vi "AI Timestamp Basics.vi"() -> ()   [LabVIEW 2020]
uses:
  <vilib>/DAQmx/write.llb/DAQmx Write (Digital Bool 1Line 1Point).vi
  <vilib>/DAQmx/read.llb/DAQmx Read (Analog Wfm 1Chan NSamp).vi
  Utility VIs/Controls/Utilities-Wait.vi/89bc9713-8f2c-40bd-a11f-1c800a437687.vi
  <vilib>/Utility/High Resolution Relative Seconds.vi
  <vilib>/DAQmx/create/channels.llb/DAQmx Create Channel (AI-Voltage-Basic).vi
  <vilib>/DAQmx/configure/timing.llb/DAQmx Timing (Sample Clock).vi
  <vilib>/DAQmx/create/channels.llb/DAQmx Create Channel (DO-Digital Output).vi
  <vilib>/Utility/High Resolution Polling Wait.vi
  <vilib>/DAQmx/miscellaneous.llb/DAQmx Fill In Error Info.vi
panel:
  out "Iteration":i32
  out "finished":bool
  out "Graph":waveform(dbl)(graph)
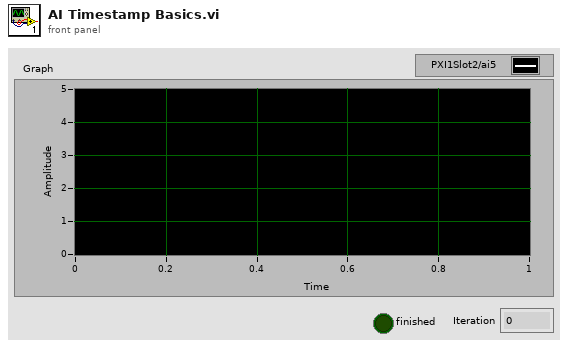
[diagram p1: front panel]
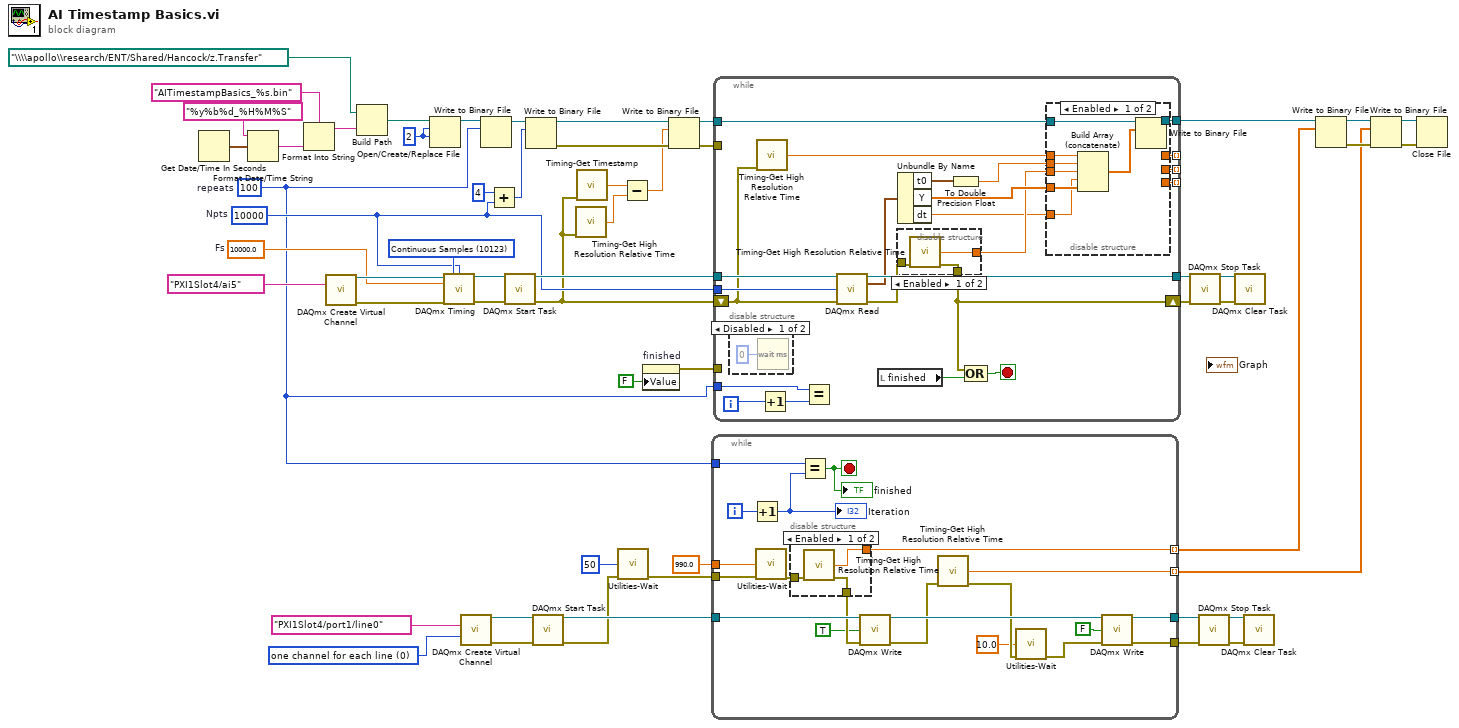
[diagram p0: block diagram]
diagram:
  w19 = 0 items=["one channel for each line", "one channel for all lines"] ("line grouping")
  w34 = u16 2
  w45 = 10000.0  # Fs
  w31 = 10000  # Npts
  w54 = 10123 items=["Finite Samples"=10178, "Continuous Samples"=10123, "Hardware Timed Single Point"=12522] ("sample mode")
  w21 = 100  # repeats
  n1 = Get Date/Time In Seconds() -> (seconds since 1Jan1904=w42:timestamp)
  n2 = Format Date/Time String(time format string (%c)="%y%b%d_%H%M%S", seconds (now)=w42) -> (date/time string=w40:string)  [unwired: 1 in]
  n3 = Format Into String(format string="AITimestampBasics_%s.bin", w40) -> (resulting string=w37:string)  [unwired: 2 in, 1 out]
  n4 = call-poly <vilib>:"DAQmx Create Virtual Channel.vi"("physical channels"=tag "PXI1Slot4/ai5") -> ("task out"=w56:refnum<k21>, "error out"=w55:errorcluster)  [unwired: 13 in]
  n5 = Build Path(base path=path "\\\\apollo\\research/ENT/Shared/Hancock/z.Transfer" ("file path (use dialog)"), name or relative path=w37) -> (appended path=w36:path)
  n6 = Open/Create/Replace File(file path (use dialog)=w36, operation (0:open)=w34, access (0:read/write)=w34) -> (refnum out=w33:refnum<file>)  [unwired: 3 in, 2 out]
  n7 = call-poly <vilib>:"DAQmx Timing.vi"("task/channels in"=w56, "sample mode"=w54, "samples per channel"=w31, "rate"=w45, "error in"=w55) -> ("task out"=w47:refnum<k21>, "error out"=w46:errorcluster)  [unwired: 9 in]
  n8 = call-poly <vilib>:"DAQmx Create Virtual Channel.vi"("lines"=tag "PXI1Slot4/port1/line0", "line grouping"=w19) -> ("task out"=w13:refnum<k21>, "error out"=w12:errorcluster)  [unwired: 12 in]
  n9 = Write to Binary File(file (use dialog)=w33, data=w21) -> (refnum out=w32:refnum<file>)  [unwired: 4 in, 2 out]
  n10 = Add(x=4, y=w31) -> (x+y=w30:i32)
  n11 = call <vilib>:"DAQmx Start Task.vi"("task/channels in"=w47, "error in"=w46) -> ("task out"=w53:refnum<k21>, "error out"=w3:errorcluster)  [unwired: 12 in]
  n12 = Write to Binary File(file (use dialog)=w32, data=w30) -> (refnum out=w27:refnum<file>, error out=w26:errorcluster)  [unwired: 4 in, 1 out]
  n13 = call <vilib>:"DAQmx Start Task.vi"("task/channels in"=w13, "error in"=w12) -> ("task out"=w14:refnum<k21>, "error out"=w10:errorcluster)  [unwired: 12 in]
  n14 = call "Timing-Get High Resolution Relative Time.vi"("error in (no error)"=w3) -> ("double precision float"=w23:dbl)  [unwired: 13 in, 1 out]
  n15 = call "Timing-Get Timestamp.vi"("error in (no error)"=w3) -> ("double precision float"=w24:dbl)  [unwired: 13 in, 1 out]
  n16 = call "Utilities-Wait.vi"("milliseconds to wait"=u32 50, "error in (no error)"=w10) -> ("error out"=w11:errorcluster)  [unwired: 13 in]
  n17 = Subtract(x=w24, y=w23) -> (x-y=w22:dbl)
  n18 = property on="finished" class="Bool (strict)"("Value"=FALSE ("finished")) -> (error out=w44:errorcluster)  [unwired: 2 in, 1 out]
  n19 = Write to Binary File(file (use dialog)=w27, data=w22, error in=w26) -> (refnum out=w28:refnum<file>, error out=w25:errorcluster)  [unwired: 3 in, 1 out]
  n20 = while {
    tunnel: w14 -> [w76]
    tunnel: [w73] -> w16
    tunnel: [w72] -> w15
    tunnel: [w70] -> w1 mode=indexing
    tunnel: w21 -> [w71]
    tunnel: [w62] -> w2 mode=indexing
    tunnel: w11 -> [w59]
    tunnel: 990.0 ("milliseconds to wait") -> [w57]
    i -> [w66]
    stop <- w67 stop-if-true
    n21 = Increment(x=w66) -> (x+1=w65:i32)
    "Iteration" <- w65
    n22 = call "Utilities-Wait.vi"("milliseconds to wait"=w57, "error in (no error)"=w59) -> ("error out"=w64:errorcluster)  [unwired: 13 in]
    n23 = disable-structure shown="Enabled" {
      disable-tunnel: w64 -> [w79 w80]
      disable-tunnel: [w78 w80] -> w63
      disable-tunnel: [w77 _] -> w62
      frame Enabled {
        n24 = call "Timing-Get High Resolution Relative Time.vi"("error in (no error)"=w79) -> ("double precision float"=w77:dbl, "error out"=w78:errorcluster)  [unwired: 13 in]
      }
      frame Disabled {
      }
    }
    n25 = Equal?(x=w71, y=w65) -> (x = y?=w67:bool)
    "finished" <- w67
    n26 = call-poly <vilib>:"DAQmx Write.vi"("task/channels in"=w76, "data"=TRUE, "error in"=w63) -> ("task out"=w75:refnum<k21>, "error out"=w69:errorcluster)  [unwired: 10 in, 1 out]
    n27 = call "Timing-Get High Resolution Relative Time.vi"("error in (no error)"=w69) -> ("double precision float"=w70:dbl, "error out"=w68:errorcluster)  [unwired: 13 in]
    n28 = call "Utilities-Wait.vi"("milliseconds to wait"=10.0, "error in (no error)"=w68) -> ("error out"=w74:errorcluster)  [unwired: 13 in]
    n29 = call-poly <vilib>:"DAQmx Write.vi"("task/channels in"=w75, "data"=FALSE, "error in"=w74) -> ("task out"=w73:refnum<k21>, "error out"=w72:errorcluster)  [unwired: 10 in, 1 out]
  }
  n30 = while {
    tunnel: w53 -> [w103]
    tunnel: [w102] -> w52
    tunnel: w31 -> [w101]
    tunnel: w44 -> [_]
    tunnel: w28 -> [w95]
    tunnel: [w94] -> w35
    tunnel: w25 -> [_]
    shift-right: [w96] -> w51
    shift-left: w3 -> [w82]
    tunnel: w21 -> [w89]
    tunnel: [w87] -> _ mode=indexing
    tunnel: [w86] -> _ mode=indexing
    tunnel: [w85] -> _ mode=indexing
    i -> [w90]
    stop <- w100 stop-if-true
    n31 = disable-structure shown="Disabled" {
      frame Disabled {
        n32 = Wait (ms)(milliseconds to wait=u32 0) -> ()  [unwired: 1 out]
      }
      frame Enabled {
      }
    }
    n33 = call "Timing-Get High Resolution Relative Time.vi"("error in (no error)"=w82) -> ("double precision float"=w81:dbl)  [unwired: 13 in, 1 out]
    n34 = Increment(x=w90) -> (x+1=w88:i32)
    n35 = Equal?(x=w89, y=w88) -> ()  [unwired: 1 out]
    n36 = call-poly <vilib>:"DAQmx Read.vi"("task/channels in"=w103, "number of samples per channel"=w101, "error in"=w82) -> ("task out"=w102:refnum<k21>, "data"=w83:waveform(dbl), "error out"=w99:errorcluster)  [unwired: 10 in]
    n37 = local read "finished"() -> (w84:bool)
    n38 = Unbundle By Name(w83) -> ("t0"=w98:timestamp, "Y"=w93:dbl[], "dt"=w91:dbl)
    n39 = disable-structure shown="Enabled" {
      disable-tunnel: w99 -> [w119 w120]
      disable-tunnel: [w118 w120] -> w96
      disable-tunnel: [w117 _] -> w92
      frame Enabled {
        n40 = call "Timing-Get High Resolution Relative Time.vi"("error in (no error)"=w119) -> ("double precision float"=w117:dbl, "error out"=w118:errorcluster)  [unwired: 13 in]
      }
      frame Disabled {
      }
    }
    n41 = To Double Precision Float(number=w98) -> (double precision float=w97:dbl)
    n42 = Compound Arithmetic op=OR(w96, w84) -> (w100:bool)
    n43 = disable-structure shown="Enabled" {
      disable-tunnel: w81 -> [w112 w115]
      disable-tunnel: w97 -> [w111 w114]
      disable-tunnel: w95 -> [w110 w116]
      disable-tunnel: [w108 w116] -> w94
      disable-tunnel: w93 -> [w107 _]
      disable-tunnel: w92 -> [w106 w113]
      disable-tunnel: w91 -> [w105 _]
      disable-tunnel: [_ w115] -> w87
      disable-tunnel: [_ w114] -> w86
      disable-tunnel: [_ w113] -> w85
      frame Enabled {
        n44 = Build Array (concatenate)(w112, w111, w106, w105, w107) -> (w109:dbl[])
        n45 = Write to Binary File(file (use dialog)=w110, data=w109) -> (refnum out=w108:refnum<file>)  [unwired: 4 in, 2 out]
      }
      frame Disabled {
      }
    }
  }
  n46 = call <vilib>:"DAQmx Stop Task.vi"("task/channels in"=w52, "error in"=w51) -> ("task out"=w50:refnum<k21>, "error out"=w49:errorcluster)  [unwired: 12 in]
  n47 = call <vilib>:"DAQmx Stop Task.vi"("task/channels in"=w16, "error in"=w15) -> ("task out"=w18:refnum<k21>, "error out"=w17:errorcluster)  [unwired: 12 in]
  n48 = call <vilib>:"DAQmx Clear Task.vi"("task in"=w50, "error in"=w49) -> ()  [unwired: 13 in, 1 out]
  n49 = call <vilib>:"DAQmx Clear Task.vi"("task in"=w18, "error in"=w17) -> ()  [unwired: 13 in, 1 out]
  n50 = Write to Binary File(file (use dialog)=w35, data=w2) -> (refnum out=w7:refnum<file>, error out=w5:errorcluster)  [unwired: 4 in, 1 out]
  n51 = Write to Binary File(file (use dialog)=w7, data=w1, error in=w5) -> (refnum out=w6:refnum<file>, error out=w4:errorcluster)  [unwired: 3 in, 1 out]
  n52 = Close File(refnum=w6, error in=w4) -> ()  [unwired: 2 out]
